vi "ClimbBegin.vi"() -> ()   [LabVIEW 2023]
uses:
  <vilib>/Rock Robotics/WPI/ThirdParty/REV Robotics/REVLib/Typedef/Spark MAX Idle Mode.ctl
  <vilib>/Rock Robotics/WPI/ThirdParty/REV Robotics/REVLib/Typedef/Spark MAX Limit Switch Polarity.ctl
  <vilib>/Rock Robotics/WPI/ThirdParty/REV Robotics/REVLib/SubVI/Public/SPARK Open Brushless.vi
  <vilib>/Rock Robotics/WPI/ThirdParty/REV Robotics/REVLib/SubVI/Public/SPARK Configure Limit Switch Forward.vi
  <vilib>/Rock Robotics/WPI/ThirdParty/REV Robotics/REVLib/SubVI/Public/SPARK Configure Limit Switch Reverse.vi
  <vilib>/Rock Robotics/WPI/ThirdParty/REV Robotics/REVLib/SubVI/Public/SPARK Configure Basic Idle Mode.vi
  <vilib>/Rock Robotics/WPI/Switch/WPI_SwitchOpenLimit.vi
  <vilib>/Rock Robotics/SystemInterfaces/DIO/FPGA_DIOChannel.ctl
panel:
  out "error out":errorcluster
  in  "error in (no error)":errorcluster
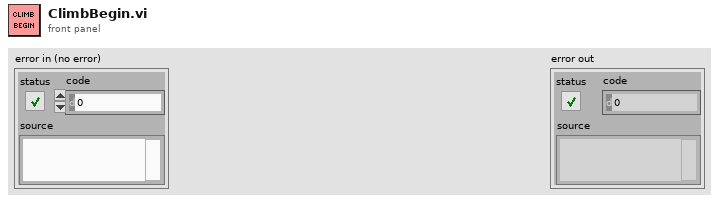
[diagram p1: front panel]
types:
  T1 = typedef "FPGA_DIOChannel.ctl" = enum8{"DIO 0", "DIO 1", "DIO 2", "DIO 3", "DIO 4", "DIO 5", "DIO 6", "DIO 7", "DIO 8", "DIO 9", "DIO MXP 0", "DIO MXP 1", "DIO MXP 2", "DIO MXP 3", "DIO MXP 4", "DIO MXP 5", "DIO MXP 6", "DIO MXP 7", "DIO MXP 8", "DIO MXP 9", "DIO MXP 10", "DIO MXP 11", "DIO MXP 12", "DIO MXP 13", "DIO MXP 14", "DIO MXP 15", "SPI Port CS1", "SPI Port CS2", "SPI Port CS3", "SPI Port MISO", "SPI Port MOSI", "Invalid"}
  T2 = typedef "Spark MAX Idle Mode.ctl" = enum16{"Coast", "Brake"}
  T3 = typedef "Spark MAX Limit Switch Polarity.ctl" = enum16{"Normally Open", "Normally Closed"}
  T4 = typedef "WPI_SwitchDevRef.ctl" = cluster{"DevStatus":errorcluster, "DIO Channel":T1, "CntIndex":T5, "Normally Closed":bool}
  T5 = typedef "FPGA_CounterCtrSystemIndex.ctl" = enum8{"Ctr 0", "Ctr 1", "Ctr 2", "Ctr 3", "Ctr 4", "Ctr 5", "Ctr 6", "Ctr 7", "Invalid"}
  T6 = typedef "WPI_MotorControlDeviceRef.ctl" = cluster{"DeviceStatus":errorcluster, "Type":T7, "PWM":cluster{"PWM Channel":T8, "DeadBand":T9}, "CAN":cluster{"Device Number":u8, "SetOutput VI Ref":variant, "GetOutput VI Ref":variant, "Enable VI Ref":variant, "Disable VI Ref":variant, "Data":variant}, "Invert":bool, "DIO PWM":cluster{"PWM \"Enable\" Channel":T8, "DIOChannel":T1, "PWM Rate":dbl}}
  T7 = typedef "WPI_MotorControlType.ctl" = enum16{"PWM", "CAN", "DIO PWM"}
  T8 = typedef "FPGA_DIOPWMChannel.ctl" = enum8{"PWM 0", "PWM 1", "PWM 2", "PWM 3", "PWM 4", "PWM 5", "PWM 6", "PWM 7", "PWM 8", "PWM 9", "PWM MXP 0", "PWM MXP 1", "PWM MXP 2", "PWM MXP 3", "PWM MXP 4", "PWM MXP 5", "PWM MXP 6", "PWM MXP 7", "PWM MXP 8", "PWM MXP 9", "Invalid"}
  T9 = typedef "WPI_PWMDeadband.ctl" = cluster{"Name":string, "maxPositivePwm":i32, "minPositivePwm":i32, "centerPwm":i32, "maxNegativePwm":i32, "minNegativePwm":i32, "angularRange":u16}
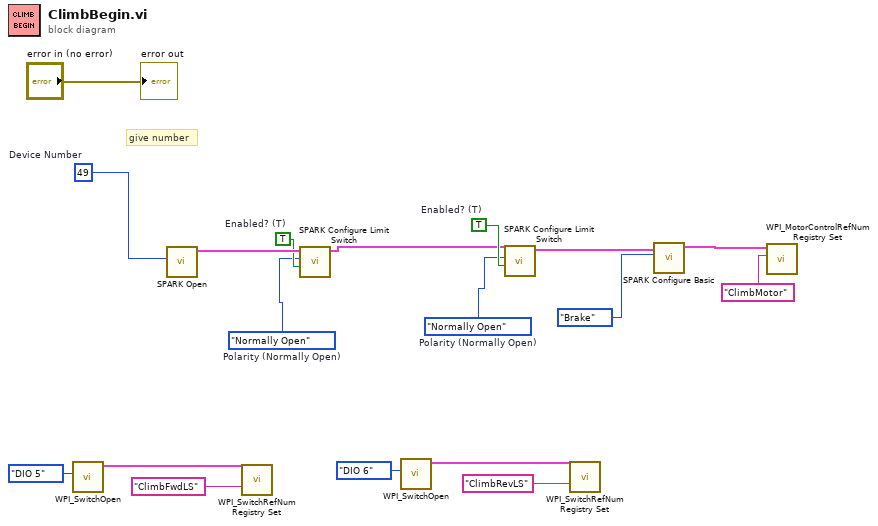
[diagram p0: block diagram]
diagram:
  w12 = Spark_MAX_Limit_Switch_Polarity."Normally Open"  # Polarity (Normally Open)
  w13 = TRUE  # Enabled? (T)
  w14 = Spark_MAX_Limit_Switch_Polarity."Normally Open"  # Polarity (Normally Open)
  w15 = TRUE  # Enabled? (T)
  w17 = u8 49  # Device Number
  # "give number"
  n1 = call-poly <vilib>:"WPI_SwitchOpen.vi"("DIO Channel"=FPGA_DIOChannel."DIO 5") -> ("SwitchDevRef"=w6:T4)  [unwired: 9 in, 1 out]
  n2 = call-poly <vilib>:"SPARK Open.vi"("Device Number"=w17) -> ("MotorControlDeviceRef"=w16:T6)  [unwired: 9 in, 1 out]
  n3 = call <vilib>:"WPI_SwitchRefNum Registry Set.vi"("refnum name"="ClimbFwdLS", "SwitchDevRef"=w6) -> ()  [unwired: 8 in, 2 out]
  n4 = call-poly <vilib>:"SPARK Configure Limit Switch.vi"("Enabled? (T)"=w15, "Polarity (Normally Open)"=w14, "MotorControlDeviceRef in"=w16) -> ("MotorControlDeviceRef out"=w11:T6)  [unwired: 7 in, 1 out]
  n5 = call-poly <vilib>:"WPI_SwitchOpen.vi"("DIO Channel"=FPGA_DIOChannel."DIO 6") -> ("SwitchDevRef"=w3:T4)  [unwired: 9 in, 1 out]
  n6 = call-poly <vilib>:"SPARK Configure Limit Switch.vi"("Enabled? (T)"=w13, "Polarity (Normally Open)"=w12, "MotorControlDeviceRef in"=w11) -> ("MotorControlDeviceRef out"=w10:T6)  [unwired: 7 in, 1 out]
  n7 = call <vilib>:"WPI_SwitchRefNum Registry Set.vi"("refnum name"="ClimbRevLS", "SwitchDevRef"=w3) -> ()  [unwired: 8 in, 2 out]
  n8 = call-poly <vilib>:"SPARK Configure Basic.vi"("Idle Mode"=Spark_MAX_Idle_Mode."Brake", "MotorControlDeviceRef in"=w10) -> ("MotorControlDeviceRef out"=w8:T6)  [unwired: 8 in, 1 out]
  n9 = call <vilib>:"WPI_MotorControlRefNum Registry Set.vi"("refnum name"="ClimbMotor", "MotorControlDevRef"=w8) -> ()  [unwired: 8 in, 2 out]
  "error out" <- "error in (no error)"
